vi "ExGetEnumInfo.vi"() -> ()   [LabVIEW 2010]
uses:
  Users/Public/Documents/SItoolkit/LabVIEW/Examples2010_5_0_0_0/Fast Examples/Open-Close Hardware/CamHandle.vi
panel:
  out "default value":dbl
  out "current value":dbl
  out "num of elements":dbl
  in  "parameter index":u32
  in  "parameter ID":u32
  out "error out":errorcluster
  in  "error in (no error)":errorcluster
  out "parameter text string":string
  out "parameter value":dbl
  out "parameter index":u32
  out "parameter ID":u32
  # "121 - vertical speed\n45 - adc speed"
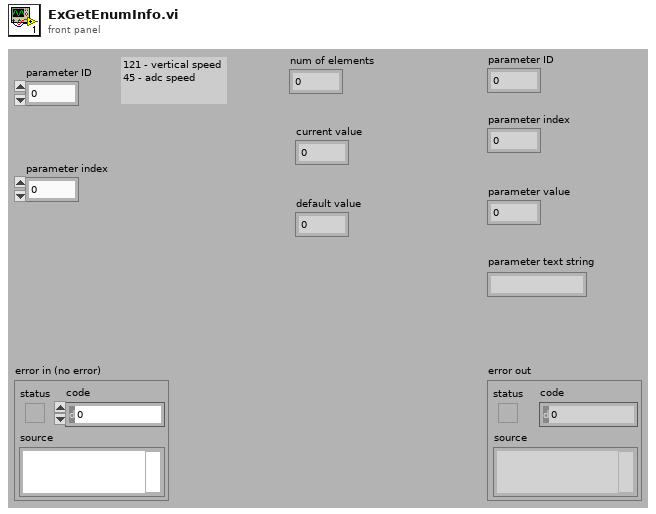
[diagram p1: front panel]
types:
  T1 = cluster{"Param ID":u32, "Avail Flag":u8, "Current Value":dbl, "Default Value":dbl, "Min Value":dbl, "Max Value":dbl, "Increment":dbl, "Data Type":u32, "Access Type":u32, "Bit Used Flag":u32, "Number of Enums":u32, "Description":string}
  T2 = cluster{"Parameter ID":u32, "Enum Index":u32, "Enum Value":dbl, "Enum String":string}
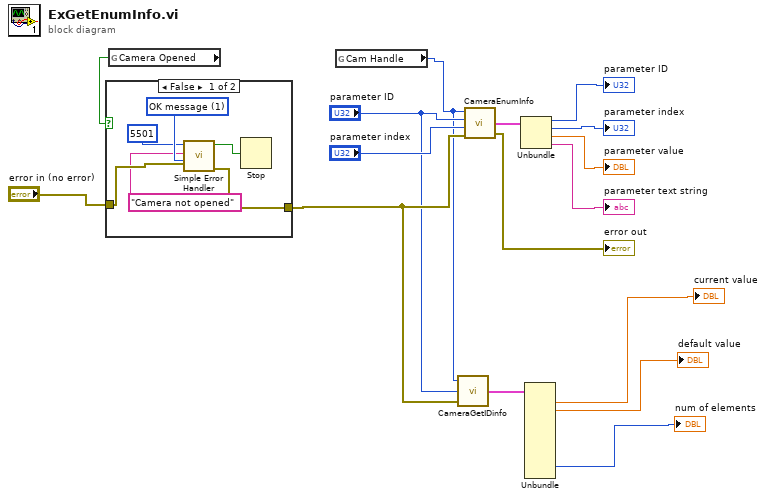
[diagram p0: block diagram]
diagram:
  n1 = global read "CamHandle.vi" "Camera Opened"() -> (w9:bool)
  n2 = case shown="False" w9 {
    tunnel: "error in (no error)" -> [w21 w23]
    tunnel: [w20 w23] -> w6
    frame False {
      w22 = u16 1 items=["no dialog", "OK message", "continue or stop message"] ("type of dialog (OK msg:1)")
      n3 = call <vilib>:"Simple Error Handler.vi"("error code (no error:0)"=5501, "error source (\" \")"="Camera not opened", "type of dialog (OK msg:1)"=w22, "error in (no error)"=w21) -> ("error?"=w18:bool, "error out"=w20:errorcluster)  [unwired: 1 in, 3 out]
      n4 = Stop(stop? (T)=w18) -> ()
    }
    frame True {
    }
  }
  n5 = global read "CamHandle.vi" "Cam Handle"() -> (w4:u32)
  n6 = call <userlib>:"CameraGetIDinfo.vi"("error in"=w6, "Param ID"="parameter ID", "Camera handle"=w4) -> ("Param ID Information"=w7:T1)  [unwired: 2 out]
  n7 = call <userlib>:"CameraEnumInfo.vi"("error in"=w6, "Enum Index"="parameter index", "Parameter ID"="parameter ID", "Camera Handle"=w4) -> ("error out"=→"error out":errorcluster, "Enum Information"=w16:T2)  [unwired: 1 out]
  n8 = Unbundle(w16) -> ("Parameter ID"=→"parameter ID":u32, "Enum Index"=→"parameter index":u32, "Enum Value"=→"parameter value":dbl, "Enum String"=→"parameter text string":string)
  n9 = Unbundle(w7) -> ("Current Value"=→"current value":dbl, "Default Value"=→"default value":dbl, "Number of Enums"=→"num of elements":u32)  [unwired: 9 out]
